vi "AttackTacticVSS.vi"(6 "State":enum16{"Exit", "GoToBall", "BallToGoal"}(ring), 8 "First call?":bool=TRUE, 9 "Game in":refnum<class "Game.lvclass">, 10 "Robot":refnum<class "Robot.lvclass">, 11 "AttackTacticVSS in":refnum<class "AttackTacticVSS.lvclass">) -> (2 "Robot out":refnum<class "Robot.lvclass">, 3 "AttackTacticVSS out":refnum<class "AttackTacticVSS.lvclass">)   [LabVIEW 2020, in "AttackTacticVSS.lvclass"]
uses:
  AttackTacticVSS.lvclass
  C:/Users/anton/Desktop/RoboIme/vsspssl/SSL_AI/Tactic_class/Tactic.lvclass
  Robot_class/Robot.lvclass
  Game_class/Game.lvclass
  Robot_class/tactics.ctl
  Tactic_class/Tactic.lvclass/Tactic.ctl
  Robot_class/Robot.lvclass/Robot.ctl
  Tactic_class/Read Skillbook.vi
  Robot_class/Write tactic.vi
  Skillbook_class/Skillbook.lvclass
  KickSkillVSS_class/KickSkillVSS.lvclass
  PenaltyPosSkillVSS_class/PenaltyPosSkillVSS.lvclass
  BallDispPosSkillVSS_class/BallDispPosSkillVSS.lvclass
  BallToGoalSkillVSS_class/BallToGoalSkillVSS.lvclass
  GoToBallSkillVSS_class/GoToBallSkillVSS.lvclass
  DefBallPosSkillVSS_class/DefBallPosSkillVSS.lvclass
  HaltSkill_class/HaltSkill.lvclass
panel:
  out "x .or. y?":bool
  out "error out 2":errorcluster
  in  "error in (no error) 2":errorcluster
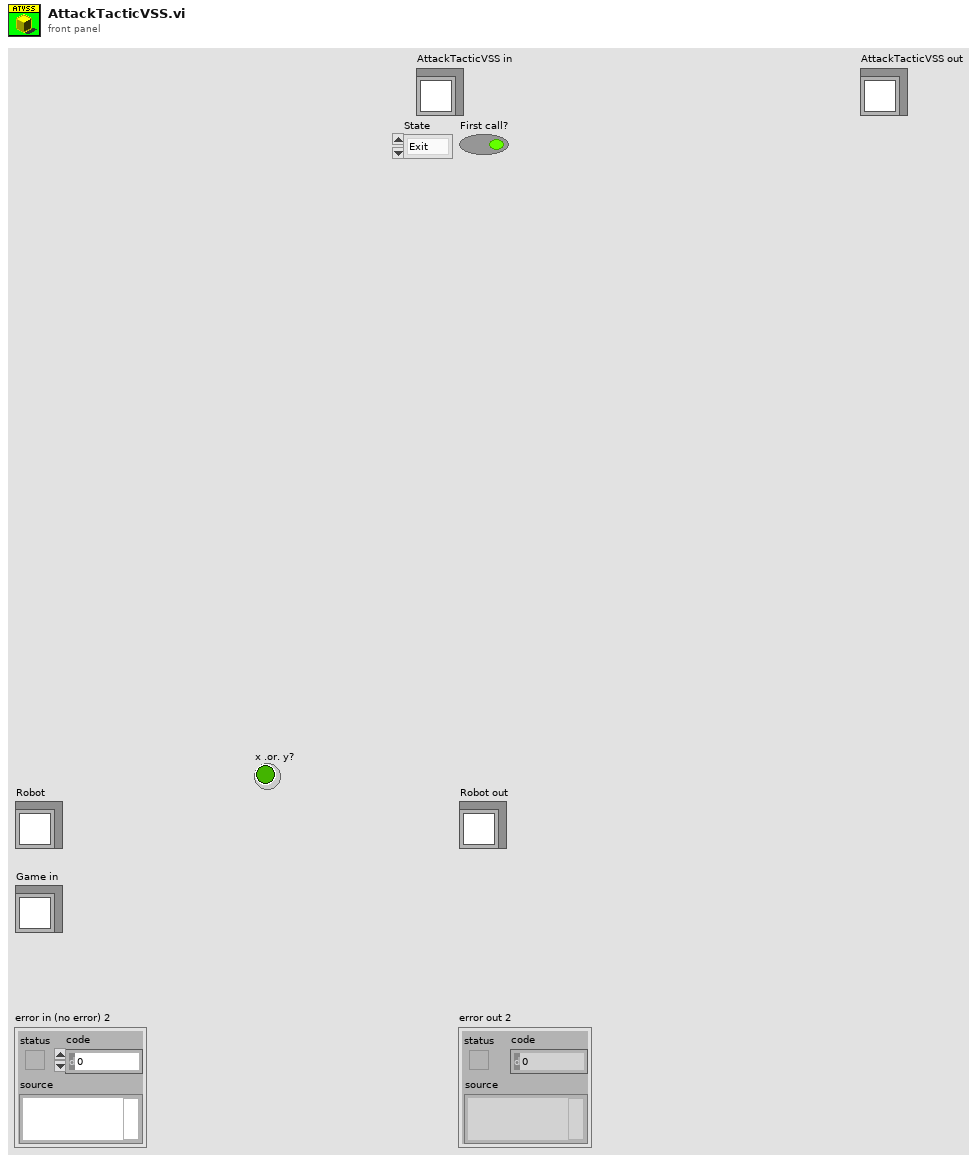
[diagram p1: front panel]
types:
  T1 = typedef "tactics.ctl" = enum16{"ReceivePassInFuturePoint", "Roller", "PrepareRollToPassRollerGoTo", "PrepareRollToPassReceiverGoTo", "WaitRoll", "PositionToRoll", "PenaltyAttacker", "PassObserver", "PenaltyDefense", "TableReceiverTactic", "Test", "DefendGoal", "Marker", "FollowAttacker", "DefendArea", "Shoot", "AttackerAimGoal", "AttackerBallOutOfField", "AttackerBlock", "AttackerStop", "Duelist", "Halt", "ZigZag", "GoTo", "Timeout", "KickToPassReceiver", "PositionToReceivePass", "DefendAreaVSS", "DefendGoalVSS", "KickVSS", "AttackVSS", "DispBallVSS", "PenaltyAttackVSS", "WaitPass"}
  T2 = cluster{"KickSkillVSS":refnum<class "KickSkillVSS.lvclass">, "PenaltyPosSkillVSS":refnum<class "PenaltyPosSkillVSS.lvclass">, "BallDispPosSkillVSS":refnum<class "BallDispPosSkillVSS.lvclass">, "BallToGoalSkillVSS":refnum<class "BallToGoalSkillVSS.lvclass">, "GoToBallSkillVSS":refnum<class "GoToBallSkillVSS.lvclass">, "DefBallPosSkillVSS":refnum<class "DefBallPosSkillVSS.lvclass">, "HaltSkill":refnum<class "HaltSkill.lvclass">}
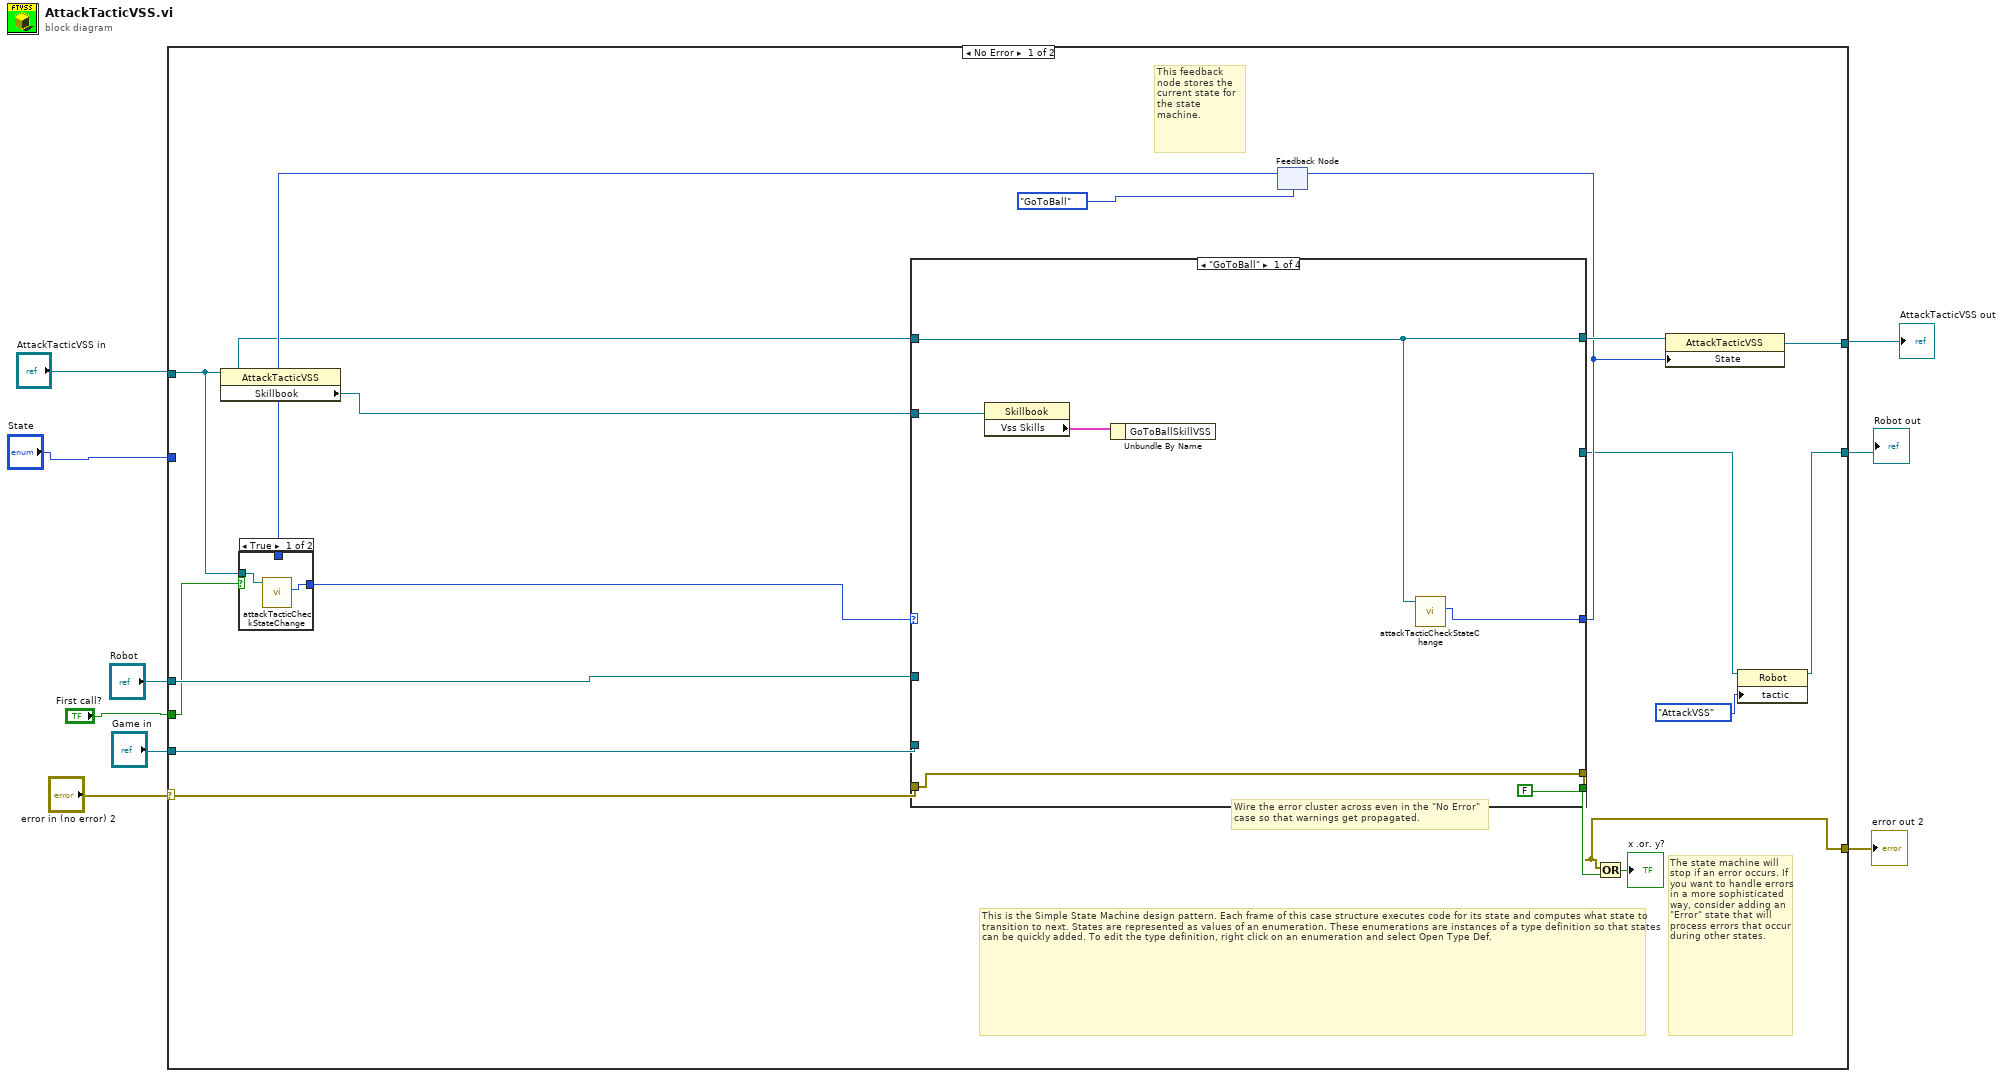
[diagram p0: block diagram]
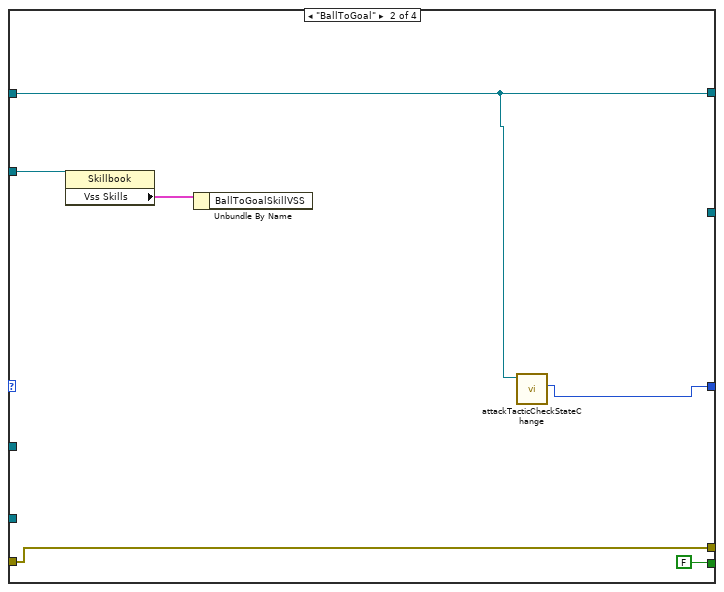
[diagram p3: hidden frame]
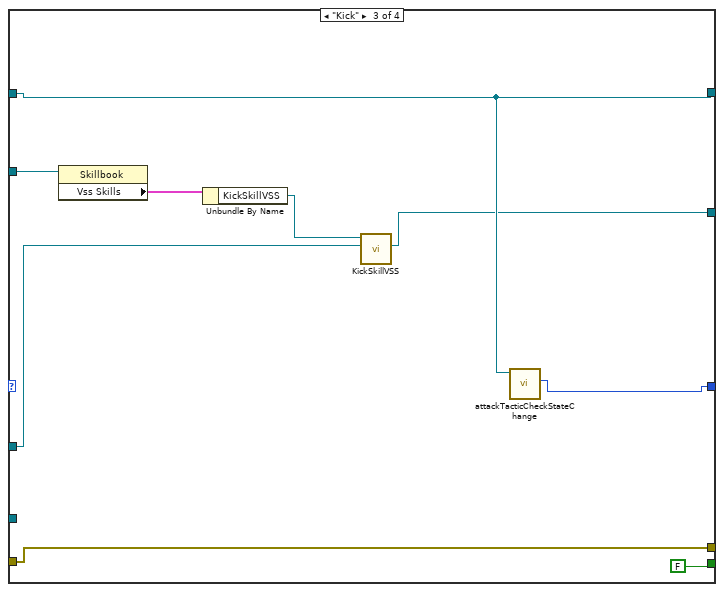
[diagram p4: hidden frame]
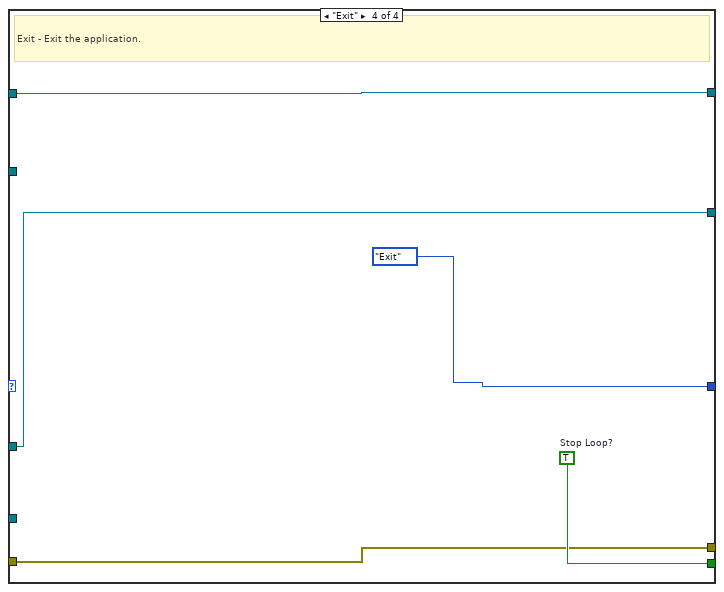
[diagram p5: hidden frame]
diagram:
  n1 = case shown="No Error" "error in (no error) 2" {
    selector: "error in (no error) 2" -> [w23 w59]
    tunnel: [w22 w59] -> w8
    tunnel: [w20 w58] -> w3
    tunnel: "AttackTacticVSS in" -> [w10 w58]
    tunnel: "Robot" -> [w15 w57]
    tunnel: "Game in" -> [w16 _]
    tunnel: [w17 w57] -> w5
    tunnel: "State" -> [_ _]
    tunnel: "First call?" -> [w14 _]
    frame No Error {
      # "The state machine will stop if an error occurs. If you want to handle errors in a more sophisticated way, consider adding an \"Error\" state that will process errors that occur during other states."
      # "This feedback node stores the current state for the state machine."
      # "This is the Simple State Machine design pattern. Each frame of this case structure executes code for its state and computes what state to transition to next. States are represented as values of an enumeration. These enumerations are instances of a type definition so that states can be quickly added. To edit the type definition, right click on an enumeration and select Open Type Def."
      # "Wire the error cluster across even in the \"No Error\"\ncase so that warnings get propagated."
      n2 = property class="AttackTacticVSS"(reference=w10) -> ("Skillbook"=w25:refnum<class "Skillbook.lvclass">)  [unwired: 1 in, 2 out]
      n3 = feedback #1(enum16{"Kick", "Exit", "GoToBall", "BallToGoal"}."GoToBall" ("State")) -> (w13:enum16{"Kick", "Exit", "GoToBall", "BallToGoal"})
      n4 = case shown="True" w14 {
        tunnel: [w29 w30] -> w12
        tunnel: w13 -> [_ w30]
        tunnel: w10 -> [w28 _]
        frame True {
          n5 = call "attackTacticCheckStateChange.vi"("AttackTacticVSS in"=w28) -> ("State"=w29:enum16{"Kick", "Exit", "GoToBall", "BallToGoal"})  [unwired: 8 in, 2 out]
        }
        frame False {
        }
      }
      n6 = case shown="\"GoToBall\"" w12 {
        tunnel: [w34 w39 w48 enum16{"Kick", "Exit", "GoToBall", "BallToGoal"}."Exit" ("State")] -> w21
        tunnel: [FALSE FALSE FALSE w56] -> w27
        tunnel: w25 -> [w35 w41 w50 _]
        tunnel: w15 -> [_ _ w44 w55]
        tunnel: [_ _ w43 w55] -> w18
        tunnel: [w33 w40 w49 w54] -> w24
        tunnel: w10 -> [w33 w40 w49 w54]
        tunnel: w16 -> [_ _ _ _]
        tunnel: [w32 w38 w46 w53] -> w22
        tunnel: w23 -> [w32 w38 w46 w53]
        frame "GoToBall" {
          n7 = property class="Skillbook"(reference=w35) -> ("Vss Skills"=w36:T2)  [unwired: 1 in, 2 out]
          n8 = Unbundle By Name(w36) -> ()  [unwired: 1 out]
          n9 = call "attackTacticCheckStateChange.vi"("AttackTacticVSS in"=w33) -> ("State"=w34:enum16{"Kick", "Exit", "GoToBall", "BallToGoal"})  [unwired: 8 in, 2 out]
        }
        frame "BallToGoal" {
          n10 = property class="Skillbook"(reference=w41) -> ("Vss Skills"=w42:T2)  [unwired: 1 in, 2 out]
          n11 = Unbundle By Name(w42) -> ()  [unwired: 1 out]
          n12 = call "attackTacticCheckStateChange.vi"("AttackTacticVSS in"=w40) -> ("State"=w39:enum16{"Kick", "Exit", "GoToBall", "BallToGoal"})  [unwired: 8 in, 2 out]
        }
        frame "Kick" {
          n13 = property class="Skillbook"(reference=w50) -> ("Vss Skills"=w51:T2)  [unwired: 1 in, 2 out]
          n14 = Unbundle By Name(w51) -> ("KickSkillVSS"=w45:refnum<class "KickSkillVSS.lvclass">)
          n15 = call-dynamic "KickSkillVSS.vi"("Robot"=w44, "KickSkillVSS in"=w45) -> ("Robot out"=w43:refnum<class "Robot.lvclass">)  [unwired: 7 in, 2 out]
          n16 = call "attackTacticCheckStateChange.vi"("AttackTacticVSS in"=w49) -> ("State"=w48:enum16{"Kick", "Exit", "GoToBall", "BallToGoal"})  [unwired: 8 in, 2 out]
        }
        frame "Exit" {
          w56 = TRUE  # Stop Loop?
          # "Exit - Exit the application."
        }
      }
      n17 = feedback-in #1(w21) -> ()
      n18 = Or(x=w22, y=w27) -> (x .or. y?=→"x .or. y?":bool)
      n19 = property class="AttackTacticVSS"(reference=w24, "State"=w21) -> (reference out=w20:refnum<class "AttackTacticVSS.lvclass">)  [unwired: 1 in, 1 out]
      n20 = property class="Robot"(reference=w18, "tactic"=tactics."AttackVSS") -> (reference out=w17:refnum<class "Robot.lvclass">)  [unwired: 1 in, 1 out]
    }
    frame Error {
    }
  }
  "AttackTacticVSS out" <- w3
  "error out 2" <- w8
  "Robot out" <- w5
